vi "Get Channel Value by Data Reference.vi"(8 "error in":errorcluster, 10 "Data Reference in":i32, 11 "VS CDAPI in":refnum<class "VS Custom Device API.lvclass">) -> (0 "error out":errorcluster, 2 "Value":dbl, 3 "VS CDAPI out":refnum<class "VS Custom Device API.lvclass">)   [LabVIEW 2026, in "Template Engine.lvlib" / "VS Custom Device API.lvclass"]
uses:
  VS Custom Device API.lvclass
  <vilib>/NI VeriStand/Custom Device API/Global Data Refs.vi
  VS Custom Device API.lvclass/VS Custom Device API.ctl
  <vilib>/NI VeriStand/Custom Device API/Custom Device API.lvlib
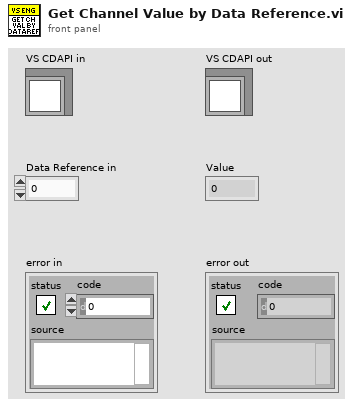
[diagram p1: front panel]
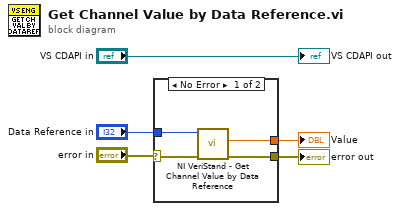
[diagram p0: block diagram]
diagram:
  n1 = case shown="No Error" "error in" {
    selector: "error in" -> [w9 w10]
    tunnel: [w8 w10] -> w3
    tunnel: "Data Reference in" -> [w7 _]
    tunnel: [w6 _] -> w1
    frame No Error {
      n2 = call <vilib>:"NI VeriStand - Get Channel Value by Data Reference.vi"("error in (no error)"=w9, "Data Reference in"=w7) -> ("error out"=w8:errorcluster, "Value"=w6:dbl)  [unwired: 8 in]
    }
    frame Error {
    }
  }
  "error out" <- w3
  "Value" <- w1
  "VS CDAPI out" <- "VS CDAPI in"
